vi "PulseGeneratorFunction-Single.vi"(1 "Ch Setup":T1={"IP Address"="192.168.126.147", "DIO #"=0, "Frequency (Hz)"=200.0, "duty cycle (%)"=0.5, "Enable"=FALSE}, 2 "Mode":T2(ring)) -> ()   [LabVIEW 2015]
uses:
  T7Examples/MODBUS/T7MOD_Write_UINT32_Register.vi
  T7Examples/MODBUS/T7MOD_Write_UINT16_Register.vi
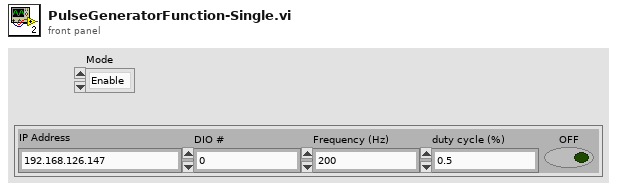
[diagram p1: front panel]
types:
  T1 = cluster{"IP Address":string, "DIO #":u16, "Frequency (Hz)":dbl, "duty cycle (%)":dbl, "Enable":bool}
  T2 = enum16{"Enable", "Disable", "Change Frequency", "Change Duty Cycle", "Configure", "Configure and Run"}
  T3 = cluster{"Clock Enable":u16, "Divisor":u16, "Roll Value":u16}
  T4 = cluster{"Pulse Enable":u16, "Index":u16, "Duty Cycle":u16}
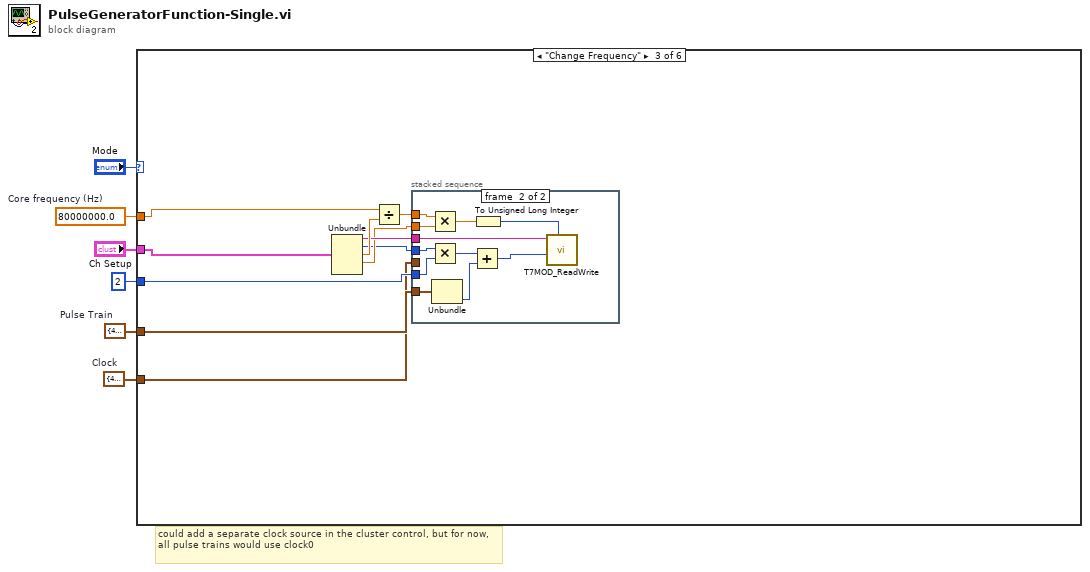
[diagram p0: block diagram]
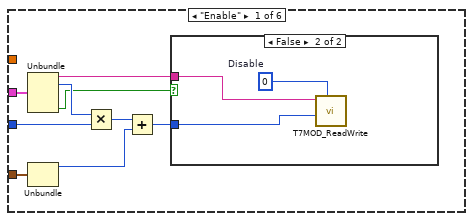
[diagram p2: hidden frame]
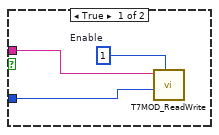
[diagram p3: hidden frame]
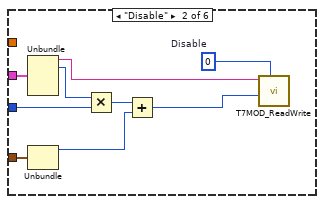
[diagram p4: hidden frame]
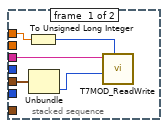
[diagram p5: hidden frame]
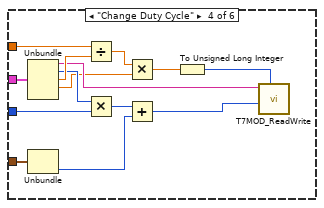
[diagram p6: hidden frame]
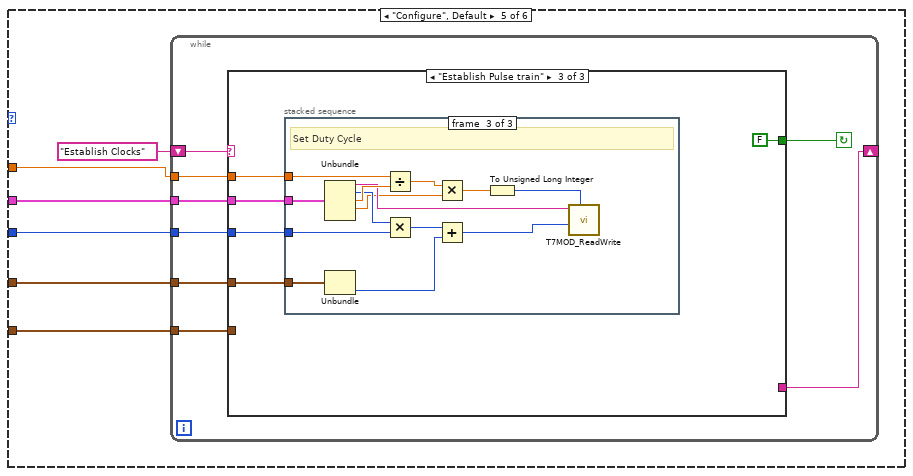
[diagram p7: hidden frame]
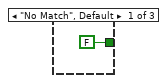
[diagram p8: hidden frame]
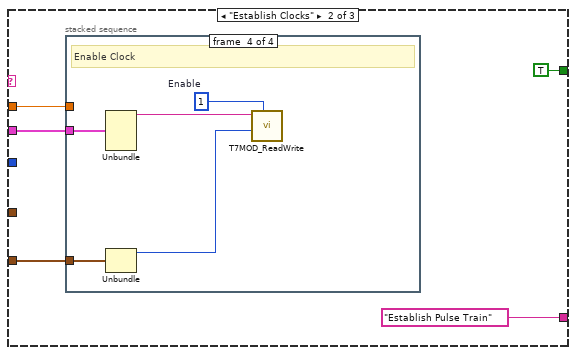
[diagram p9: hidden frame]
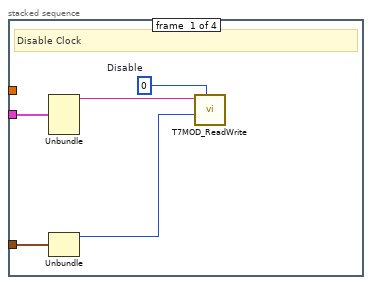
[diagram p10: hidden frame]
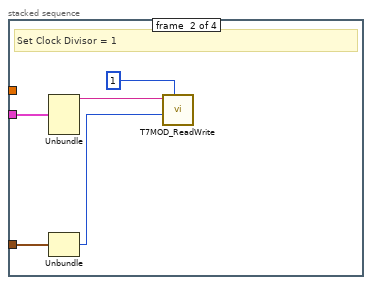
[diagram p11: hidden frame]
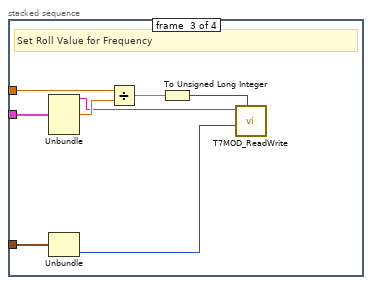
[diagram p12: hidden frame]
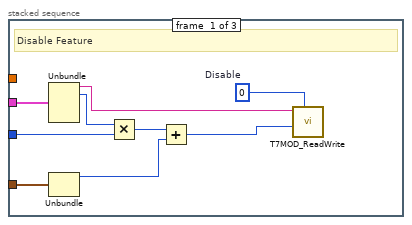
[diagram p13: hidden frame]
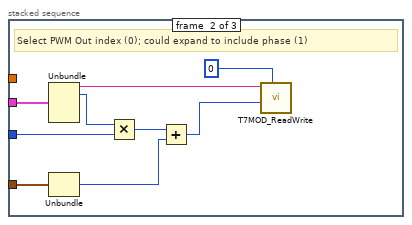
[diagram p14: hidden frame]
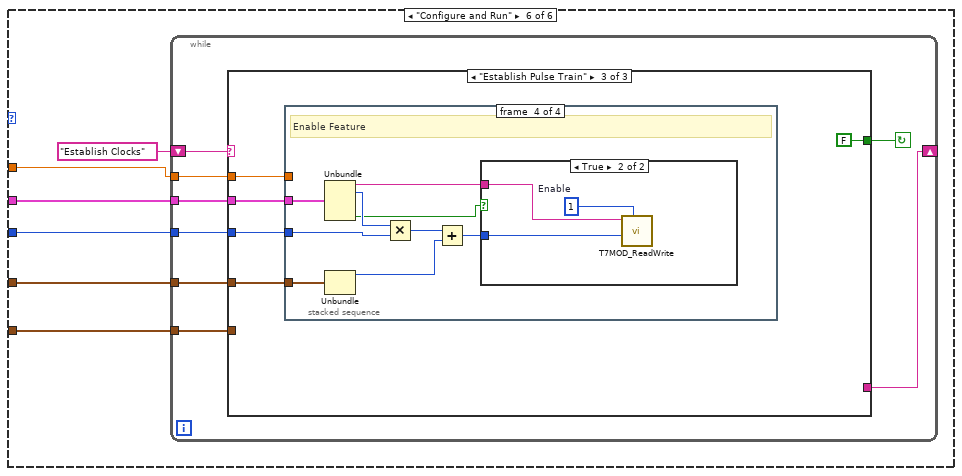
[diagram p15: hidden frame]
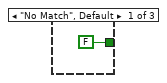
[diagram p16: hidden frame]
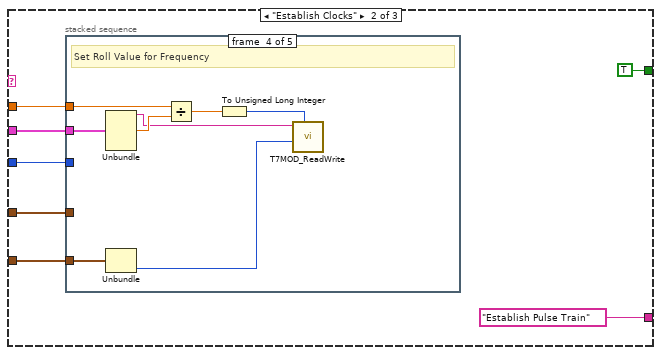
[diagram p17: hidden frame]
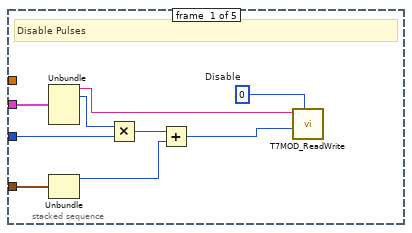
[diagram p18: hidden frame]
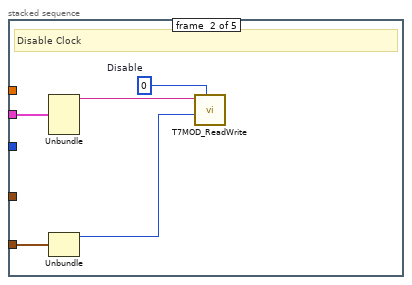
[diagram p19: hidden frame]
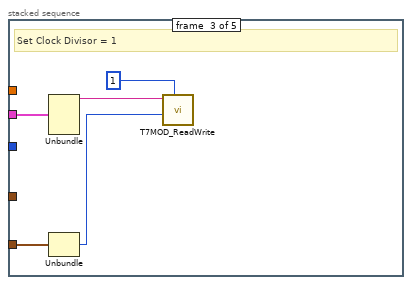
[diagram p20: hidden frame]
diagram:
  w2 = T3 {"Clock Enable"=44900, "Divisor"=44901, "Roll Value"=44904}  # Clock
  w3 = T4 {"Pulse Enable"=44000, "Index"=44100, "Duty Cycle"=44300}  # Pulse Train
  w5 = 80000000.0  # Core frequency (Hz)
  # "could add a separate clock source in the cluster control, but for now, all pulse trains would use clock0"
  n1 = case shown="\"Change Frequency\"" "Mode" {
    tunnel: "Ch Setup" -> [w15 w30 w35 w70 w76 w156]
    tunnel: w5 -> [_ _ w40 w69 w74 w154]
    tunnel: 2 -> [w14 w29 w34 w68 w73 w153]
    tunnel: w3 -> [w13 w28 w36 w67 w72 w152]
    tunnel: w2 -> [_ _ w31 _ w71 w151]
    frame "Enable" {
      n2 = Unbundle(w15) -> ("IP Address"=w8:string, "DIO #"=w12:u16, "Enable"=w7:bool)  [unwired: 2 out]
      n3 = Unbundle(w13) -> ("Pulse Enable"=w10:u16)  [unwired: 2 out]
      n4 = Multiply(x=w12, y=w14) -> (x*y=w11:i32)
      n5 = Add(x=w11, y=w10) -> (x+y=w9:i32)
      n6 = case shown="False" w7 {
        tunnel: w9 -> [w18 w21]
        tunnel: w8 -> [w17 w20]
        frame True {
          w16 = u32 1  # Enable
          n7 = call-poly "T7MOD_ReadWrite.vi"("UINT32 to Write"=w16, "LabJack UINT32 Register"=w18, "Remote IP Address"=w17) -> ()  [unwired: 7 in, 2 out]
        }
        frame False {
          w19 = u32 0  # Disable
          n8 = call-poly "T7MOD_ReadWrite.vi"("UINT32 to Write"=w19, "LabJack UINT32 Register"=w21, "Remote IP Address"=w20) -> ()  [unwired: 7 in, 2 out]
        }
      }
    }
    frame "Disable" {
      w22 = u32 0  # Disable
      n9 = Unbundle(w30) -> ("IP Address"=w23:string, "DIO #"=w27:u16)  [unwired: 3 out]
      n10 = Unbundle(w28) -> ("Pulse Enable"=w25:u16)  [unwired: 2 out]
      n11 = Multiply(x=w27, y=w29) -> (x*y=w26:i32)
      n12 = Add(x=w26, y=w25) -> (x+y=w24:i32)
      n13 = call-poly "T7MOD_ReadWrite.vi"("UINT32 to Write"=w22, "LabJack UINT32 Register"=w24, "Remote IP Address"=w23) -> ()  [unwired: 7 in, 2 out]
    }
    frame "Change Frequency" {
      n14 = Unbundle(w35) -> ("IP Address"=w37:string, "DIO #"=w32:u16, "Frequency (Hz)"=w39:dbl, "duty cycle (%)"=w33:dbl)  [unwired: 1 out]
      n15 = Divide(x=w40, y=w39) -> (x/y=w38:dbl)
      n16 = stacked-sequence {
        tunnel: w38 -> [w45 w50]
        tunnel: w37 -> [w43 w49]
        tunnel: w36 -> [_ w51]
        tunnel: w34 -> [_ w48]
        tunnel: w33 -> [_ w47]
        tunnel: w32 -> [_ w46]
        tunnel: w31 -> [w42 _]
        frame #0 {
          n17 = To Unsigned Long Integer(number=w45) -> (unsigned 32bit integer=w44:u32)
          n18 = Unbundle(w42) -> ("Roll Value"=w41:u16)  [unwired: 2 out]
          n19 = call-poly "T7MOD_ReadWrite.vi"("UINT32 to Write"=w44, "LabJack UINT32 Register"=w41, "Remote IP Address"=w43) -> ()  [unwired: 7 in, 2 out]
        }
        frame #1 {
          n20 = Multiply(x=w50, y=w47) -> (x*y=w52:dbl)
          n21 = Multiply(x=w46, y=w48) -> (x*y=w56:i32)
          n22 = Unbundle(w51) -> ("Duty Cycle"=w55:u16)  [unwired: 2 out]
          n23 = Add(x=w56, y=w55) -> (x+y=w53:i32)
          n24 = To Unsigned Long Integer(number=w52) -> (unsigned 32bit integer=w54:u32)
          n25 = call-poly "T7MOD_ReadWrite.vi"("UINT32 to Write"=w54, "LabJack UINT32 Register"=w53, "Remote IP Address"=w49) -> ()  [unwired: 7 in, 2 out]
        }
      }
    }
    frame "Change Duty Cycle" {
      n26 = Unbundle(w70) -> ("IP Address"=w60:string, "DIO #"=w65:u16, "Frequency (Hz)"=w66:dbl, "duty cycle (%)"=w57:dbl)  [unwired: 1 out]
      n27 = Unbundle(w67) -> ("Duty Cycle"=w63:u16)  [unwired: 2 out]
      n28 = Divide(x=w69, y=w66) -> (x/y=w58:dbl)
      n29 = Multiply(x=w65, y=w68) -> (x*y=w64:i32)
      n30 = Multiply(x=w58, y=w57) -> (x*y=w59:dbl)
      n31 = Add(x=w64, y=w63) -> (x+y=w61:i32)
      n32 = To Unsigned Long Integer(number=w59) -> (unsigned 32bit integer=w62:u32)
      n33 = call-poly "T7MOD_ReadWrite.vi"("UINT32 to Write"=w62, "LabJack UINT32 Register"=w61, "Remote IP Address"=w60) -> ()  [unwired: 7 in, 2 out]
    }
    frame "Configure", Default {
      n34 = while {
        tunnel: w74 -> [w83]
        tunnel: w71 -> [w82]
        tunnel: w76 -> [w81]
        tunnel: w72 -> [w80]
        tunnel: w73 -> [w79]
        shift-right: [w78] -> _
        shift-left: "Establish Clocks" -> [w84]
        stop <- w77 continue-if-true
        n35 = case shown="\"Establish Pulse train\"" w84 {
          tunnel: w81 -> [_ w90 w118]
          tunnel: w83 -> [_ w89 w117]
          tunnel: w82 -> [_ w88 _]
          tunnel: w80 -> [_ _ w116]
          tunnel: w79 -> [_ _ w115]
          tunnel: [_ "Establish Pulse Train" _] -> w78
          tunnel: [FALSE TRUE FALSE] -> w77
          frame "No Match", Default {
          }
          frame "Establish Clocks" {
            n36 = stacked-sequence {
              tunnel: w90 -> [w91 w96 w101 w109]
              tunnel: w89 -> [_ _ w108 _]
              tunnel: w88 -> [w95 w100 w107 w113]
              frame #0 {
                w92 = u16 0  # Disable
                # "Disable Clock"
                n37 = Unbundle(w91) -> ("IP Address"=w93:string)  [unwired: 4 out]
                n38 = Unbundle(w95) -> ("Clock Enable"=w94:u16)  [unwired: 2 out]
                n39 = call-poly "T7MOD_ReadWrite.vi"("UINT16 to Write"=w92, "LabJack UINT16 Register"=w94, "Remote IP Address"=w93) -> ()  [unwired: 7 in, 2 out]
              }
              frame #1 {
                # "Set Clock Divisor = 1"
                n40 = Unbundle(w96) -> ("IP Address"=w99:string)  [unwired: 4 out]
                n41 = Unbundle(w100) -> ("Divisor"=w97:u16)  [unwired: 2 out]
                n42 = call-poly "T7MOD_ReadWrite.vi"("UINT16 to Write"=u16 1 ("Disable"), "LabJack UINT16 Register"=w97, "Remote IP Address"=w99) -> ()  [unwired: 7 in, 2 out]
              }
              frame #2 {
                # "Set Roll Value for Frequency"
                n43 = Unbundle(w101) -> ("IP Address"=w102:string, "Frequency (Hz)"=w106:dbl)  [unwired: 3 out]
                n44 = Unbundle(w107) -> ("Roll Value"=w104:u16)  [unwired: 2 out]
                n45 = Divide(x=w108, y=w106) -> (x/y=w105:dbl)
                n46 = To Unsigned Long Integer(number=w105) -> (unsigned 32bit integer=w103:u32)
                n47 = call-poly "T7MOD_ReadWrite.vi"("UINT32 to Write"=w103, "LabJack UINT32 Register"=w104, "Remote IP Address"=w102) -> ()  [unwired: 7 in, 2 out]
              }
              frame #3 {
                w110 = u16 1  # Enable
                # "Enable Clock"
                n48 = Unbundle(w109) -> ("IP Address"=w111:string)  [unwired: 4 out]
                n49 = Unbundle(w113) -> ("Clock Enable"=w112:u16)  [unwired: 2 out]
                n50 = call-poly "T7MOD_ReadWrite.vi"("UINT16 to Write"=w110, "LabJack UINT16 Register"=w112, "Remote IP Address"=w111) -> ()  [unwired: 7 in, 2 out]
              }
            }
          }
          frame "Establish Pulse train" {
            n51 = stacked-sequence {
              tunnel: w118 -> [w127 w136 w150]
              tunnel: w117 -> [_ _ w149]
              tunnel: w116 -> [w126 w135 w148]
              tunnel: w115 -> [w125 w134 w147]
              frame #0 {
                w119 = u32 0  # Disable
                # "Disable Feature"
                n52 = Unbundle(w127) -> ("IP Address"=w120:string, "DIO #"=w124:u16)  [unwired: 3 out]
                n53 = Unbundle(w126) -> ("Pulse Enable"=w122:u16)  [unwired: 2 out]
                n54 = Multiply(x=w124, y=w125) -> (x*y=w123:i32)
                n55 = Add(x=w123, y=w122) -> (x+y=w121:i32)
                n56 = call-poly "T7MOD_ReadWrite.vi"("UINT32 to Write"=w119, "LabJack UINT32 Register"=w121, "Remote IP Address"=w120) -> ()  [unwired: 7 in, 2 out]
              }
              frame #1 {
                # "Select PWM Out index (0); could expand to include phase (1)"
                n57 = Unbundle(w136) -> ("IP Address"=w130:string, "DIO #"=w133:u16)  [unwired: 3 out]
                n58 = Unbundle(w135) -> ("Index"=w128:u16)  [unwired: 2 out]
                n59 = Multiply(x=w133, y=w134) -> (x*y=w132:i32)
                n60 = Add(x=w132, y=w128) -> (x+y=w131:i32)
                n61 = call-poly "T7MOD_ReadWrite.vi"("UINT32 to Write"=u32 0 ("Disable"), "LabJack UINT32 Register"=w131, "Remote IP Address"=w130) -> ()  [unwired: 7 in, 2 out]
              }
              frame #2 {
                # "Set Duty Cycle"
                n62 = Unbundle(w150) -> ("IP Address"=w140:string, "DIO #"=w145:u16, "Frequency (Hz)"=w146:dbl, "duty cycle (%)"=w137:dbl)  [unwired: 1 out]
                n63 = Unbundle(w148) -> ("Duty Cycle"=w143:u16)  [unwired: 2 out]
                n64 = Divide(x=w149, y=w146) -> (x/y=w138:dbl)
                n65 = Multiply(x=w145, y=w147) -> (x*y=w144:i32)
                n66 = Multiply(x=w138, y=w137) -> (x*y=w139:dbl)
                n67 = Add(x=w144, y=w143) -> (x+y=w141:i32)
                n68 = To Unsigned Long Integer(number=w139) -> (unsigned 32bit integer=w142:u32)
                n69 = call-poly "T7MOD_ReadWrite.vi"("UINT32 to Write"=w142, "LabJack UINT32 Register"=w141, "Remote IP Address"=w140) -> ()  [unwired: 7 in, 2 out]
              }
            }
          }
        }
      }
    }
    frame "Configure and Run" {
      n70 = while {
        tunnel: w154 -> [w163]
        tunnel: w151 -> [w162]
        tunnel: w156 -> [w161]
        tunnel: w152 -> [w160]
        tunnel: w153 -> [w159]
        shift-right: [w158] -> _
        shift-left: "Establish Clocks" -> [w164]
        stop <- w157 continue-if-true
        n71 = case shown="\"Establish Pulse Train\"" w164 {
          tunnel: w161 -> [_ w172 w209]
          tunnel: w163 -> [_ w171 w208]
          tunnel: w162 -> [_ w170 _]
          tunnel: w160 -> [_ w167 w207]
          tunnel: w159 -> [_ w166 w206]
          tunnel: [_ "Establish Pulse Train" _] -> w158
          tunnel: [FALSE TRUE FALSE] -> w157
          frame "No Match", Default {
          }
          frame "Establish Clocks" {
            n72 = stacked-sequence {
              tunnel: w172 -> [w181 w182 w187 w192 w200]
              tunnel: w171 -> [_ _ _ w199 _]
              tunnel: w170 -> [_ w186 w191 w198 w204]
              tunnel: w167 -> [w180 _ _ _ _]
              tunnel: w166 -> [w179 _ _ _ _]
              frame #0 {
                w173 = u32 0  # Disable
                # "Disable Pulses"
                n73 = Unbundle(w181) -> ("IP Address"=w174:string, "DIO #"=w178:u16)  [unwired: 3 out]
                n74 = Unbundle(w180) -> ("Pulse Enable"=w176:u16)  [unwired: 2 out]
                n75 = Multiply(x=w178, y=w179) -> (x*y=w177:i32)
                n76 = Add(x=w177, y=w176) -> (x+y=w175:i32)
                n77 = call-poly "T7MOD_ReadWrite.vi"("UINT32 to Write"=w173, "LabJack UINT32 Register"=w175, "Remote IP Address"=w174) -> ()  [unwired: 7 in, 2 out]
              }
              frame #1 {
                w183 = u16 0  # Disable
                # "Disable Clock"
                n78 = Unbundle(w182) -> ("IP Address"=w184:string)  [unwired: 4 out]
                n79 = Unbundle(w186) -> ("Clock Enable"=w185:u16)  [unwired: 2 out]
                n80 = call-poly "T7MOD_ReadWrite.vi"("UINT16 to Write"=w183, "LabJack UINT16 Register"=w185, "Remote IP Address"=w184) -> ()  [unwired: 7 in, 2 out]
              }
              frame #2 {
                # "Set Clock Divisor = 1"
                n81 = Unbundle(w187) -> ("IP Address"=w190:string)  [unwired: 4 out]
                n82 = Unbundle(w191) -> ("Divisor"=w188:u16)  [unwired: 2 out]
                n83 = call-poly "T7MOD_ReadWrite.vi"("UINT16 to Write"=u16 1 ("Disable"), "LabJack UINT16 Register"=w188, "Remote IP Address"=w190) -> ()  [unwired: 7 in, 2 out]
              }
              frame #3 {
                # "Set Roll Value for Frequency"
                n84 = Unbundle(w192) -> ("IP Address"=w193:string, "Frequency (Hz)"=w197:dbl)  [unwired: 3 out]
                n85 = Unbundle(w198) -> ("Roll Value"=w195:u16)  [unwired: 2 out]
                n86 = Divide(x=w199, y=w197) -> (x/y=w196:dbl)
                n87 = To Unsigned Long Integer(number=w196) -> (unsigned 32bit integer=w194:u32)
                n88 = call-poly "T7MOD_ReadWrite.vi"("UINT32 to Write"=w194, "LabJack UINT32 Register"=w195, "Remote IP Address"=w193) -> ()  [unwired: 7 in, 2 out]
              }
              frame #4 {
                w201 = u16 1  # Enable
                # "Enable Clock"
                n89 = Unbundle(w200) -> ("IP Address"=w202:string)  [unwired: 4 out]
                n90 = Unbundle(w204) -> ("Clock Enable"=w203:u16)  [unwired: 2 out]
                n91 = call-poly "T7MOD_ReadWrite.vi"("UINT16 to Write"=w201, "LabJack UINT16 Register"=w203, "Remote IP Address"=w202) -> ()  [unwired: 7 in, 2 out]
              }
            }
          }
          frame "Establish Pulse Train" {
            n92 = stacked-sequence {
              tunnel: w209 -> [w218 w227 w241 w250]
              tunnel: w208 -> [_ _ w240 _]
              tunnel: w207 -> [w217 w226 w239 w249]
              tunnel: w206 -> [w216 w225 w238 w248]
              frame #0 {
                w210 = u32 0  # Disable
                # "Disable Feature"
                n93 = Unbundle(w218) -> ("IP Address"=w211:string, "DIO #"=w215:u16)  [unwired: 3 out]
                n94 = Unbundle(w217) -> ("Pulse Enable"=w213:u16)  [unwired: 2 out]
                n95 = Multiply(x=w215, y=w216) -> (x*y=w214:i32)
                n96 = Add(x=w214, y=w213) -> (x+y=w212:i32)
                n97 = call-poly "T7MOD_ReadWrite.vi"("UINT32 to Write"=w210, "LabJack UINT32 Register"=w212, "Remote IP Address"=w211) -> ()  [unwired: 7 in, 2 out]
              }
              frame #1 {
                # "Select PWM Out index (0); could expand to include phase (1)"
                n98 = Unbundle(w227) -> ("IP Address"=w221:string, "DIO #"=w224:u16)  [unwired: 3 out]
                n99 = Unbundle(w226) -> ("Index"=w219:u16)  [unwired: 2 out]
                n100 = Multiply(x=w224, y=w225) -> (x*y=w223:i32)
                n101 = Add(x=w223, y=w219) -> (x+y=w222:i32)
                n102 = call-poly "T7MOD_ReadWrite.vi"("UINT32 to Write"=u32 0 ("Disable"), "LabJack UINT32 Register"=w222, "Remote IP Address"=w221) -> ()  [unwired: 7 in, 2 out]
              }
              frame #2 {
                # "Set Duty Cycle"
                n103 = Unbundle(w241) -> ("IP Address"=w231:string, "DIO #"=w236:u16, "Frequency (Hz)"=w237:dbl, "duty cycle (%)"=w228:dbl)  [unwired: 1 out]
                n104 = Unbundle(w239) -> ("Duty Cycle"=w234:u16)  [unwired: 2 out]
                n105 = Divide(x=w240, y=w237) -> (x/y=w229:dbl)
                n106 = Multiply(x=w236, y=w238) -> (x*y=w235:i32)
                n107 = Multiply(x=w229, y=w228) -> (x*y=w230:dbl)
                n108 = Add(x=w235, y=w234) -> (x+y=w232:i32)
                n109 = To Unsigned Long Integer(number=w230) -> (unsigned 32bit integer=w233:u32)
                n110 = call-poly "T7MOD_ReadWrite.vi"("UINT32 to Write"=w233, "LabJack UINT32 Register"=w232, "Remote IP Address"=w231) -> ()  [unwired: 7 in, 2 out]
              }
              frame #3 {
                # "Enable Feature"
                n111 = Unbundle(w250) -> ("IP Address"=w243:string, "DIO #"=w247:u16, "Enable"=w242:bool)  [unwired: 2 out]
                n112 = Unbundle(w249) -> ("Pulse Enable"=w245:u16)  [unwired: 2 out]
                n113 = Multiply(x=w247, y=w248) -> (x*y=w246:i32)
                n114 = Add(x=w246, y=w245) -> (x+y=w244:i32)
                n115 = case shown="True" w242 {
                  tunnel: w244 -> [_ w253]
                  tunnel: w243 -> [_ w252]
                  frame False {
                  }
                  frame True {
                    w251 = u32 1  # Enable
                    n116 = call-poly "T7MOD_ReadWrite.vi"("UINT32 to Write"=w251, "LabJack UINT32 Register"=w253, "Remote IP Address"=w252) -> ()  [unwired: 7 in, 2 out]
                  }
                }
              }
            }
          }
        }
      }
    }
  }
